vi "Lockin.DAQ.Simulate Noisy AI.vi"(4 "Simulate Waveguide [T]":bool=TRUE, 6 "Waveguide Cluster":T1={"Vsource Index"=0, "Vsg Index"=1, "V+"=0, "V-"=0}, 8 "error in (no error)":errorcluster, 10 "AO []":waveform(dbl)[](array[waveform]), 11 "Lockin.DAQ in":refnum<class "Lockin.DAQ.lvclass">) -> (0 "error out":errorcluster, 2 "Noisy AI []":waveform(dbl)[](array[waveform]), 3 "Lockin.DAQ out":refnum<class "Lockin.DAQ.lvclass">)   [LabVIEW 2016, in "Lockin.DAQ.lvclass"]
uses:
  Lockin.DAQ.lvclass
  Waveguide Model/Waveguide Model--Cluster.ctl
  Lockin.DAQ.lvclass/Lockin.DAQ.ctl
  <vilib>/Analysis/2dsp.llb/Real FFT.vi
  <vilib>/Analysis/2dsp.llb/Inverse Real FFT.vi
  <vilib>/Analysis/2dsp.llb/Decimate (single shot).vi
  <vilib>/Analysis/2dsp.llb/Decimate (single shot, DBL).vi
  <vilib>/Utility/High Resolution Relative Seconds.vi
  <vilib>/Waveform/WDTOps.llb/Number of Waveform Samples.vi
  <vilib>/Waveform/WDTOps.llb/WDT Number of Waveform Samples DBL.vi
  <vilib>/Utility/error.llb/Error Cluster From Error Code.vi
  <vilib>/measure/NI_MABase.lvlib
  <vilib>/Analysis/NI_AALPro.lvlib
panel:
  in  "Noise Cluster":T2={"1/f vs. Uniform "=1.0, "60Hz Amplitude"=0.005, "Gauss/Unif %"=0.5, "Noise Amp"=0.005}
  out "Signal Graph":waveform(dbl)[](graph)
  out "Noisy Signal Graph":waveform(dbl)[](graph)
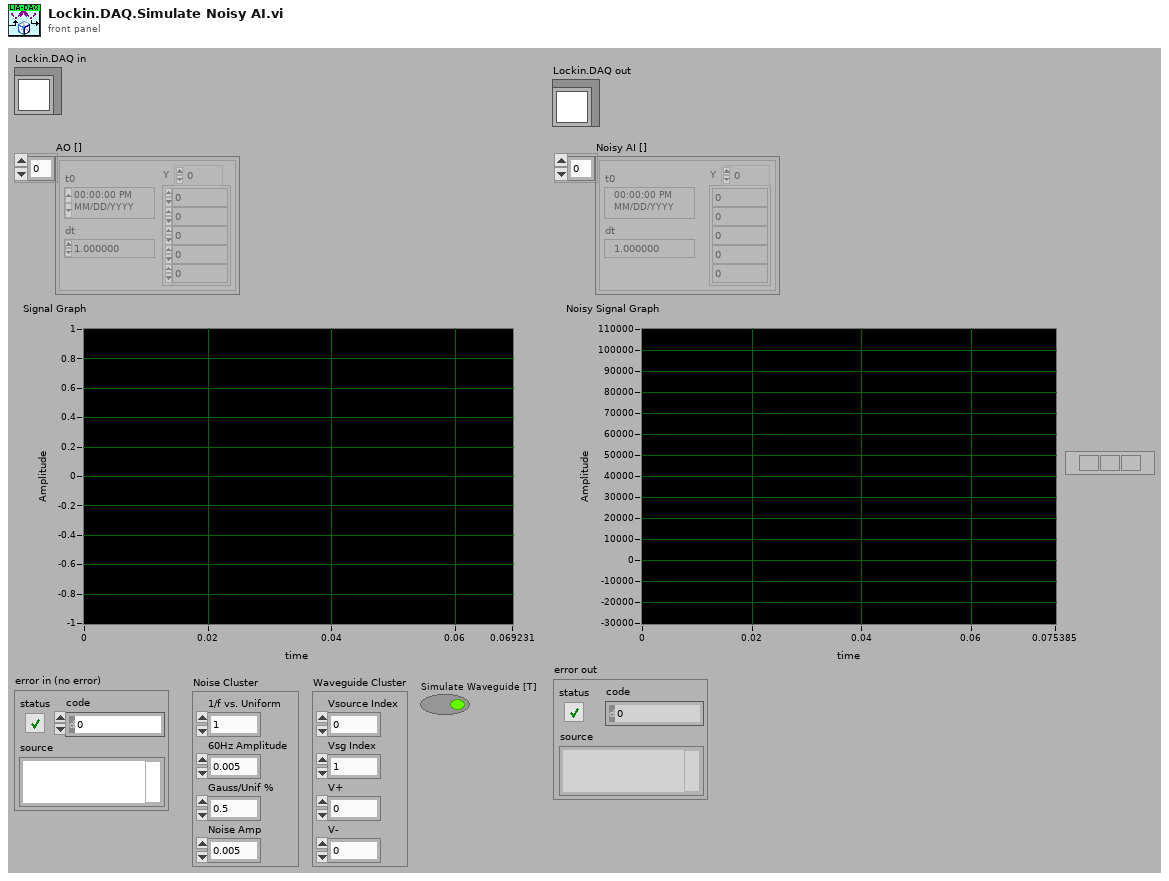
[diagram p1: front panel]
types:
  T1 = typedef "Lockin.DAQ.lvclass/Waveguide Model--Cluster.ctl" = cluster{"Vsource Index":i32, "Vsg Index":i32, "V+":i32, "V-":i32}
  T2 = cluster{"1/f vs. Uniform ":dbl, "60Hz Amplitude":dbl, "Gauss/Unif %":dbl, "Noise Amp":dbl}
  T3 = typedef "Lockin.DAQ.lvclass/AI Simulation-enum.ctl" = enum16{"AI = HW simulated", "AI = noise*AO", "AI = waveguide"}
  T4 = typedef "Lockin.DAQ.lvclass/Sampling.ctl" = cluster{"Fs":dbl, "#s":i32}
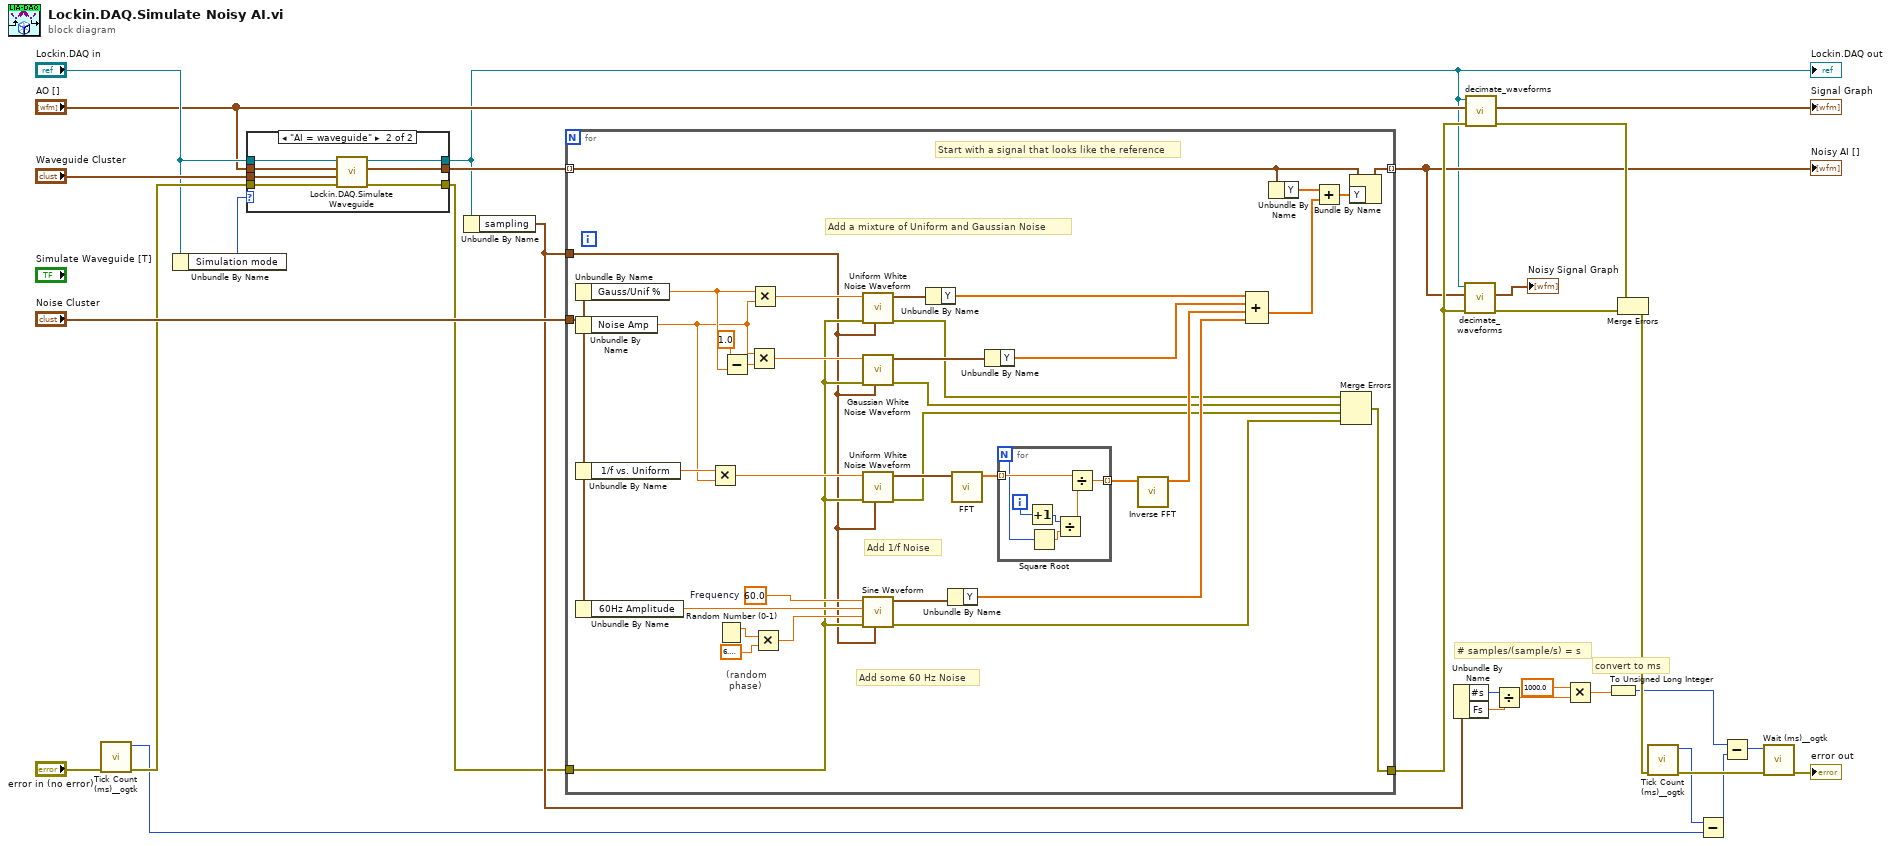
[diagram p0: block diagram]
diagram:
  # "convert to ms"
  # "# samples/(sample/s) = s"
  n1 = call <userlib>:"Tick Count (ms)__ogtk.vi"("error in (no error)"="error in (no error)") -> ("error out"=w13:errorcluster, "millisecond timer value"=w7:u32)  [unwired: 9 in]
  n2 = Unbundle By Name("Lockin.DAQ in") -> ("Simulation mode"=w3:T3)
  n3 = case shown="\"AI = waveguide\"" w3 {
    tunnel: w13 -> [w32 w40]
    tunnel: [w32 w39] -> w4
    tunnel: [w31 w38] -> w9
    tunnel: "Waveguide Cluster" -> [_ w37]
    tunnel: "AO []" -> [w31 w36]
    tunnel: "Lockin.DAQ in" -> [w33 w35]
    tunnel: [w33 w34] -> w1
    frame "AI = noise*AO", Default {
    }
    frame "AI = waveguide" {
      n4 = call "Lockin.DAQ.Simulate Waveguide.vi"("error in (no error)"=w40, "Waveguide Cluster"=w37, "AO []"=w36, "Lockin.DAQ in"=w35) -> ("error out"=w39:errorcluster, "AI []"=w38:waveform(dbl)[], "Lockin.DAQ out"=w34:refnum<class "Lockin.DAQ.lvclass">)  [unwired: 5 in]
    }
  }
  "Lockin.DAQ out" <- w1
  n5 = Unbundle By Name(w1) -> ("sampling"=w8:T4)
  n6 = for {
    tunnel: "Noise Cluster" -> [w56]
    tunnel: w8 -> [w45]
    tunnel: [w46] -> w6 mode=indexing
    tunnel: w4 -> [w50]
    tunnel: [w47] -> w29
    tunnel: w9 -> [w41] mode=indexing
    w51 = 60.0  # Frequency
    # "Start with a signal that looks like the reference"
    # "Add 1/f Noise"
    # "(random\n phase)"
    # "Add some 60 Hz Noise"
    # "Add a mixture of Uniform and Gaussian Noise"
    n7 = Unbundle By Name(w56) -> ("Gauss/Unif %"=w61:dbl)
    n8 = Unbundle By Name(w56) -> ("Noise Amp"=w42:dbl)
    n9 = Unbundle By Name(w56) -> ("1/f vs. Uniform"=w60:dbl)
    n10 = Unbundle By Name(w56) -> ("60Hz Amplitude"=w59:dbl)
    n11 = Multiply(x=w60, y=w42) -> (x*y=w67:dbl)
    n12 = Random Number (0-1)() -> (number: 0 to 1=w71:dbl)
    n13 = Subtract(x=1.0, y=w61) -> (x-y=w74:dbl)
    n14 = Multiply(x=w42, y=w74) -> (x*y=w55:dbl)
    n15 = Multiply(x=w61, y=w42) -> (x*y=w54:dbl)
    n16 = Multiply(x=w71, y=6.283185307179586) -> (x*y=w53:dbl)
    n17 = call <vilib>:"Uniform White Noise Waveform.vi"("sampling info"=w45, "error in (no error)"=w50, "amplitude"=w54) -> ("error out"=w43:errorcluster, "signal out"=w75:waveform(dbl))  [unwired: 7 in]
    n18 = call <vilib>:"Gaussian White Noise Waveform.vi"("sampling info"=w45, "error in (no error)"=w50, "standard deviation"=w55) -> ("error out"=w44:errorcluster, "signal out"=w76:waveform(dbl))  [unwired: 7 in]
    n19 = call <vilib>:"Uniform White Noise Waveform.vi"("sampling info"=w45, "error in (no error)"=w50, "amplitude"=w67) -> ("error out"=w49:errorcluster, "signal out"=w66:waveform(dbl))  [unwired: 7 in]
    n20 = call <vilib>:"Sine Waveform.vi"("sampling info"=w45, "error in (no error)"=w50, "phase"=w53, "amplitude"=w59, "frequency"=w51) -> ("error out"=w48:errorcluster, "signal out"=w70:waveform(dbl))  [unwired: 5 in]
    n21 = Unbundle By Name(w75) -> ("Y"=w69:dbl[])
    n22 = Unbundle By Name(w70) -> ("Y"=w65:dbl[])
    n23 = call-poly <vilib>:"FFT.vi"("X"=w66) -> ("FFT {X}"=w52:cdb[])  [unwired: 9 in, 1 out]
    n24 = Unbundle By Name(w76) -> ("Y"=w62:dbl[])
    n25 = for {
      N -> [w80]
      tunnel: [w83] -> w68 mode=indexing
      tunnel: w52 -> [w82] mode=indexing
      i -> [w81]
      n26 = Increment(x=w81) -> (x+1=w78:i32)
      n27 = Square Root(x=w80) -> (sqrt(x)=w79:dbl)
      n28 = Divide(x=w78, y=w79) -> (x/y=w77:dbl)
      n29 = Divide(x=w82, y=w77) -> (x/y=w83:cdb)
    }
    n30 = call-poly <vilib>:"Inverse FFT.vi"("FFT {X}"=w68) -> ("X"=w64:dbl[])  [unwired: 9 in, 1 out]
    n31 = Compound Arithmetic op=ADD(w69, w62, w64, w65) -> (w63:dbl[])
    n32 = Unbundle By Name(w41) -> ("Y"=w58:dbl[])
    n33 = Add(x=w58, y=w63) -> (x+y=w57:dbl[])
    n34 = Merge Errors(w43, w44, w49, w48) -> (w47:errorcluster)
    n35 = Bundle By Name(cluster=w41, "Y"=w57) -> (w46:waveform(dbl))
  }
  "Noisy AI []" <- w6
  n36 = Unbundle By Name(w8) -> ("#s"=w16:i32, "Fs"=w17:dbl)
  n37 = call "decimate_waveforms.vi"("error in (no error)"=w29, "WFM"=w6, "LockinDAQ"=w1) -> ("error out"=w28:errorcluster, "WFM out"=→"Noisy Signal Graph":waveform(dbl)[])  [unwired: 6 in, 1 out]
  n38 = call "decimate_waveforms.vi"("error in (no error)"=w29, "WFM"="AO []", "LockinDAQ"=w1) -> ("error out"=w27:errorcluster, "WFM out"=→"Signal Graph":waveform(dbl)[])  [unwired: 6 in, 1 out]
  n39 = Divide(x=w16, y=w17) -> (x/y=w20:dbl)
  n40 = Multiply(x=1000.0, y=w20) -> (x*y=w19:dbl)
  n41 = To Unsigned Long Integer(number=w19) -> (unsigned 32bit integer=w15:u32)
  n42 = Merge Errors(w27, w28) -> (w26:errorcluster)
  n43 = call <userlib>:"Tick Count (ms)__ogtk.vi"("error in (no error)"=w26) -> ("error out"=w25:errorcluster, "millisecond timer value"=w21:u32)  [unwired: 9 in]
  n44 = Subtract(x=w21, y=w7) -> (x-y=w22:u32)
  n45 = Subtract(x=w15, y=w22) -> (x-y=w23:u32)
  n46 = call <userlib>:"Wait (ms)__ogtk.vi"("error in (no error)"=w25, "milliseconds to wait"=w23) -> ("error out"=→"error out":errorcluster)  [unwired: 8 in, 1 out]
